vi "Configure Active DUT Control Automation Framework.vi"(8 "error in (no error)":errorcluster, 10 "Control Automation Framework (External Automation Application)":i32(ring) items=["External Automation Application"], 11 "VISA resource name":refnum<visa-resource-name>) -> (0 "error out":errorcluster, 3 "VISA resource name out":refnum<visa-resource-name>)   [LabVIEW 2020, in "Rohde&Schwarz CMXP Base.lvlib"]
doc: "Selects the type of automation.\n\nAttribute:\nRSCMXPBASE_ATTR_ACTIVE_DUT_CONTROL_AUTOMATION_FRAMEWORK\n\nRemote-control command:\n[CONFigure:]DUT:CONTrol:AUTO:FRAMework"
uses:
  <instrlib>/Rohde&Schwarz CMXP Base/Rohde&Schwarz CMXP Base.lvlib
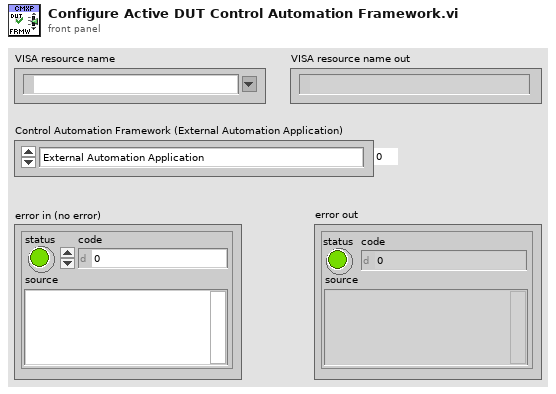
[diagram p1: front panel]
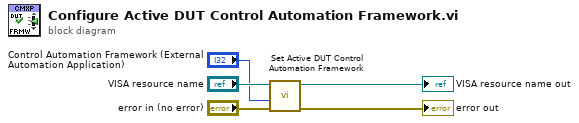
[diagram p0: block diagram]
diagram:
  n1 = call "Set Active DUT Control Automation Framework"("error in (no error)"="error in (no error)", "Active DUT Control Automation Framework (0 - External Automation Application)"="Control Automation Framework (External Automation Application)", "instrument handle"="VISA resource name") -> ("error out"=→"error out":errorcluster, "instrument handle out"=→"VISA resource name out":refnum<visa-resource-name>)  [unwired: 7 in]
